vi "TPG261_ReadPressure.vi"(8 "error in (no error)":errorcluster caption="Fehler (Eingang, kein Fehler)", 11 "input refnum":refnum<visa-resource-name> caption="ComPort") -> (0 "error out":errorcluster, 2 "Pressure Sensor 1":dbl format="%.3e")   [LabVIEW 2012]
doc: "This VI is an example of how to use the PV ActiveLine subVIs programmatically. This VI first initializes the instrument, takes measurements, then closes the instrument."
uses:
  <instrlib>/PV ActiveLine/PV ActiveLine.lvlib
panel:
  out "Status Sensor 1":i32(ring) items=["data OK", "underrange", "overrange", "sensor error", "sensor off", "no sensor", "ID error"]
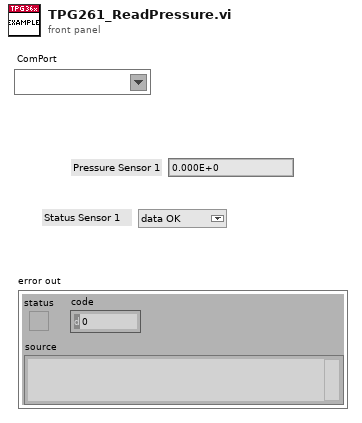
[diagram p1: front panel]
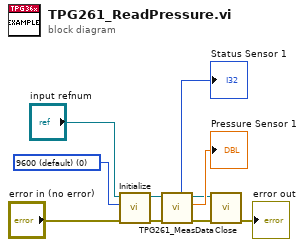
[diagram p0: block diagram]
diagram:
  w7 = u32 0 items=["9600 (default)", "19200", "38400", "57600", "115200"] ("Baud Rate")
  n1 = call <instrlib>:"Initialize.vi"("error in (no error)"="error in (no error)", "Baud Rate"=w7, "input refnum"="input refnum") -> ("Cluster (Ausgang)"=w6:errorcluster, "Referenz out"=w5:refnum<visa-resource-name>)  [unwired: 7 in]
  n2 = call "TPG261_MeasData.vi"("Fehler (Eingang)"=w6, "Referenz in"=w5) -> ("Cluster (Ausgang)"=w2:errorcluster, "Pressure CH1"=→"Pressure Sensor 1":dbl, "Referenz out"=w1:refnum<visa-resource-name>, "Status CH1"=→"Status Sensor 1":i32)  [unwired: 6 in]
  n3 = call <instrlib>:"Close.vi"("error in (no error)"=w2, "VISA resource name"=w1) -> ("error out"=→"error out":errorcluster)  [unwired: 9 in]
